vi "test Float Writes to Source.vi"(8 "error in (no error)":errorcluster, 11 "TestCase in":refnum<class "Parameter Setting.lvclass">) -> (0 "error out":errorcluster, 3 "TestCase out":refnum<class "Parameter Setting.lvclass">)   [LabVIEW 2017, in "Deterministic Error Tests.lvlib" / "Parameter Setting.lvclass"]
uses:
  Parameter Setting.lvclass
  Parameter Setting.lvclass/Parameter Setting.ctl
  Source/VIs/VIs for Poly/Write SGL into Source.vi
  Source/VIs/VIs for Poly/Write DBL into Source.vi
  <vilib>/addons/_JKI Toolkits/VI Tester/TestCase.llb/TestCase.lvclass
  Source/Deterministic Error Builder.lvlib
  C:/Program Files (x86)/National Instruments/LabVIEW 2017/vi.lib/addons/_JKI Toolkits/VI Tester/TestCase.llb/TestCase.lvclass
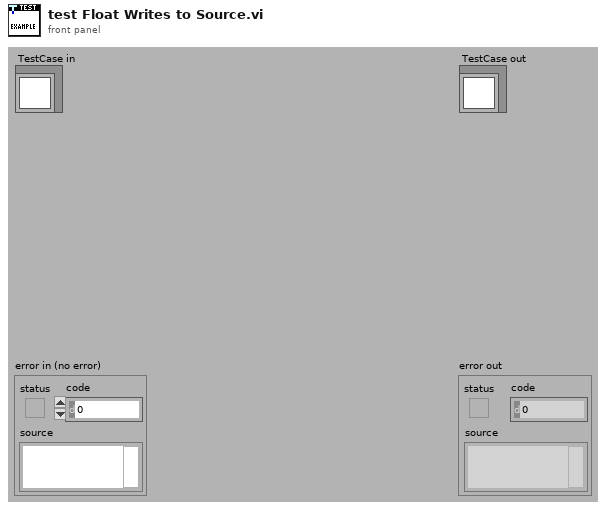
[diagram p1: front panel]
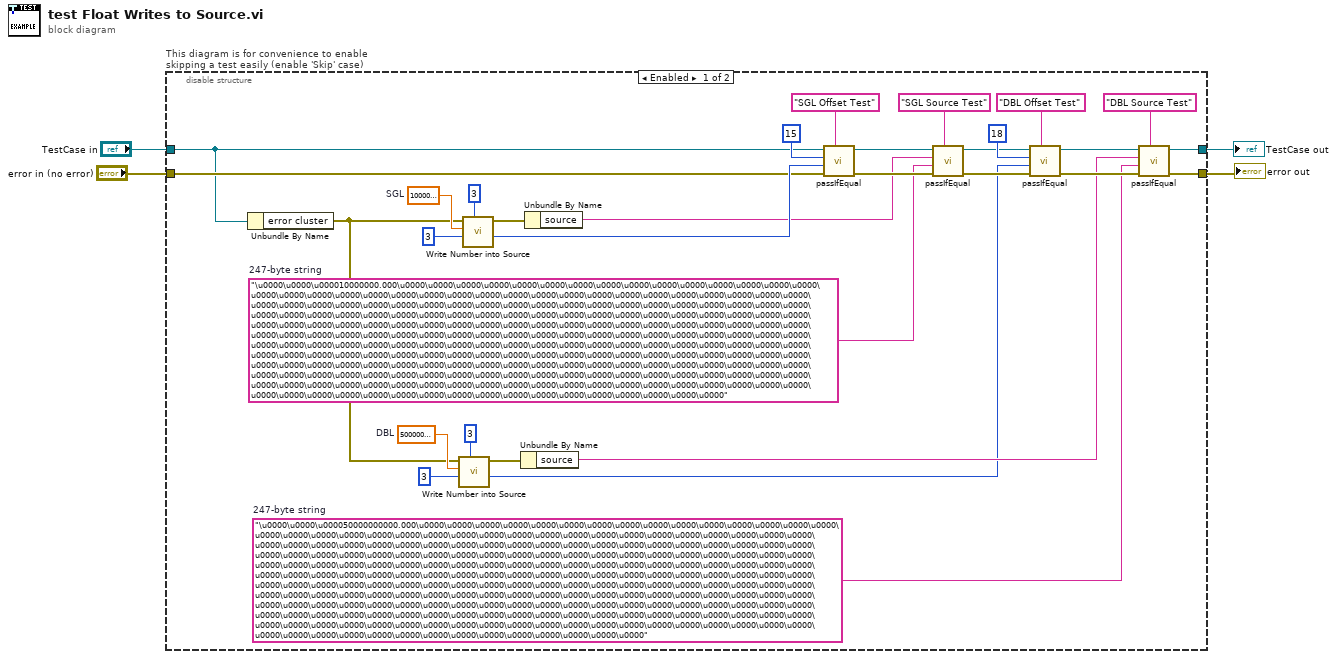
[diagram p0: block diagram]
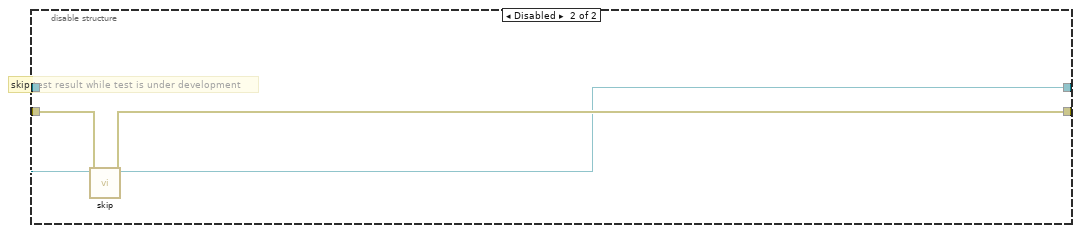
[diagram p2: hidden frame]
diagram:
  n1 = disable-structure "This diagram is for convenience to enable skipping a test easily (enable 'Skip' case)" shown="Enabled" {
    disable-tunnel: "TestCase in" -> [w7 w39]
    disable-tunnel: [w9 w37] -> w1
    disable-tunnel: [w5 w38] -> w3
    disable-tunnel: "error in (no error)" -> [w8 w36]
    frame Enabled {
      w10 = "\u0000\u0000\u000050000000000.000\u0000\u0000\u0000\u0000\u0000\u0000\u0000\u0000\u0000\u0000\u0000\u0000\u0000\u0000\u0000\u0000\u0000\u0000\u0000\u0000\u0000\u0000\u0000\u0000\u0000\u0000\u0000\u0000\u0000\u0000\u0000\u0000\u0000\u0000\u0000\u0000\u0000\u0000\u0000\u0000\u0000\u0000\u0000\u0000\u0000\u0000\u0000\u0000\u0000\u0000\u0000\u0000\u0000\u0000\u0000\u0000\u0000\u0000\u0000\u0000\u0000\u0000\u0000\u0000\u0000\u0000\u0000\u0000\u0000\u0000\u0000\u0000\u0000\u0000\u0000\u0000\u0000\u0000\u0000\u0000\u0000\u0000\u0000\u0000\u0000\u0000\u0000\u0000\u0000\u0000\u0000\u0000\u0000\u0000\u0000\u0000\u0000\u0000\u0000\u0000\u0000\u0000\u0000\u0000\u0000\u0000\u0000\u0000\u0000\u0000\u0000\u0000\u0000\u0000\u0000\u0000\u0000\u0000\u0000\u0000\u0000\u0000\u0000\u0000\u0000\u0000\u0000\u0000\u0000\u0000\u0000\u0000\u0000\u0000\u0000\u0000\u0000\u0000\u0000\u0000\u0000\u0000\u0000\u0000\u0000\u0000\u0000\u0000\u0000\u0000\u0000\u0000\u0000\u0000\u0000\u0000\u0000\u0000\u0000\u0000\u0000\u0000\u0000\u0000\u0000\u0000\u0000\u0000\u0000\u0000\u0000\u0000\u0000\u0000\u0000\u0000\u0000\u0000\u0000\u0000\u0000\u0000\u0000\u0000\u0000\u0000\u0000\u0000\u0000\u0000\u0000\u0000\u0000\u0000\u0000\u0000\u0000\u0000\u0000\u0000\u0000\u0000\u0000\u0000\u0000\u0000\u0000\u0000\u0000\u0000\u0000\u0000\u0000\u0000\u0000\u0000\u0000\u0000\u0000\u0000\u0000\u0000\u0000\u0000\u0000\u0000\u0000\u0000\u0000"  # 247-byte string
      w20 = 50000000000.0  # DBL
      w25 = "\u0000\u0000\u000010000000.000\u0000\u0000\u0000\u0000\u0000\u0000\u0000\u0000\u0000\u0000\u0000\u0000\u0000\u0000\u0000\u0000\u0000\u0000\u0000\u0000\u0000\u0000\u0000\u0000\u0000\u0000\u0000\u0000\u0000\u0000\u0000\u0000\u0000\u0000\u0000\u0000\u0000\u0000\u0000\u0000\u0000\u0000\u0000\u0000\u0000\u0000\u0000\u0000\u0000\u0000\u0000\u0000\u0000\u0000\u0000\u0000\u0000\u0000\u0000\u0000\u0000\u0000\u0000\u0000\u0000\u0000\u0000\u0000\u0000\u0000\u0000\u0000\u0000\u0000\u0000\u0000\u0000\u0000\u0000\u0000\u0000\u0000\u0000\u0000\u0000\u0000\u0000\u0000\u0000\u0000\u0000\u0000\u0000\u0000\u0000\u0000\u0000\u0000\u0000\u0000\u0000\u0000\u0000\u0000\u0000\u0000\u0000\u0000\u0000\u0000\u0000\u0000\u0000\u0000\u0000\u0000\u0000\u0000\u0000\u0000\u0000\u0000\u0000\u0000\u0000\u0000\u0000\u0000\u0000\u0000\u0000\u0000\u0000\u0000\u0000\u0000\u0000\u0000\u0000\u0000\u0000\u0000\u0000\u0000\u0000\u0000\u0000\u0000\u0000\u0000\u0000\u0000\u0000\u0000\u0000\u0000\u0000\u0000\u0000\u0000\u0000\u0000\u0000\u0000\u0000\u0000\u0000\u0000\u0000\u0000\u0000\u0000\u0000\u0000\u0000\u0000\u0000\u0000\u0000\u0000\u0000\u0000\u0000\u0000\u0000\u0000\u0000\u0000\u0000\u0000\u0000\u0000\u0000\u0000\u0000\u0000\u0000\u0000\u0000\u0000\u0000\u0000\u0000\u0000\u0000\u0000\u0000\u0000\u0000\u0000\u0000\u0000\u0000\u0000\u0000\u0000\u0000\u0000\u0000\u0000\u0000\u0000\u0000\u0000\u0000\u0000\u0000\u0000\u0000\u0000\u0000\u0000"  # 247-byte string
      w30 = sgl 10000000.0  # SGL
      n2 = Unbundle By Name(w7) -> ("error cluster"=w6:errorcluster)
      n3 = call-poly "Write Number into Source.vi"("precision (3)"=i16 3, "offset"=3, "value"=w20, "error in"=w6) -> ("new offset"=w11:i32, "error out"=w22:errorcluster)  [unwired: 6 in]
      n4 = call-poly "Write Number into Source.vi"("precision (3)"=i16 3, "offset"=3, "value"=w30, "error in"=w6) -> ("new offset"=w27:i32, "error out"=w28:errorcluster)  [unwired: 6 in]
      n5 = Unbundle By Name(w22) -> ("source"=w12:string)
      n6 = Unbundle By Name(w28) -> ("source"=w26:string)
      n7 = call-dynamic "passIfEqual.vi"("custom report message (\"\")"="SGL Offset Test" ("custom report message (\"\")"), "error in (no error)"=w8, "y"=w27, "x"=15 ("offset"), "TestCase in"=w7) -> ("error out"=w31:errorcluster, "TestCase out"=w32:refnum<class "Parameter Setting.lvclass">)  [unwired: 5 in]
      n8 = call-dynamic "passIfEqual.vi"("custom report message (\"\")"="SGL Source Test" ("custom report message (\"\")"), "error in (no error)"=w31, "y"=w25, "x"=w26, "TestCase in"=w32) -> ("error out"=w15:errorcluster, "TestCase out"=w16:refnum<class "Parameter Setting.lvclass">)  [unwired: 5 in]
      n9 = call-dynamic "passIfEqual.vi"("custom report message (\"\")"="DBL Offset Test" ("custom report message (\"\")"), "error in (no error)"=w15, "y"=w11, "x"=18 ("offset"), "TestCase in"=w16) -> ("error out"=w13:errorcluster, "TestCase out"=w19:refnum<class "Parameter Setting.lvclass">)  [unwired: 5 in]
      n10 = call-dynamic "passIfEqual.vi"("custom report message (\"\")"="DBL Source Test" ("custom report message (\"\")"), "error in (no error)"=w13, "y"=w10, "x"=w12, "TestCase in"=w19) -> ("error out"=w5:errorcluster, "TestCase out"=w9:refnum<class "Parameter Setting.lvclass">)  [unwired: 5 in]
    }
    frame Disabled {
      # "skip test result while test is under development"
      n11 = call <vilib>:"skip.vi"("error in (no error)"=w36, "TestCase in"=w39) -> ("error out"=w38:errorcluster, "TestCase out"=w37:refnum<class "Parameter Setting.lvclass">)  [unwired: 8 in]
    }
  }
  "error out" <- w3
  "TestCase out" <- w1
